vi "PopupViewLastErrorMessage.vi"() -> ()   [LabVIEW 2010]
uses:
  030 - EVENTS/03 - ToMessageHandlerProcess/enumMessageCriticity.ctl
  030 - EVENTS/EnumFgvEventCommand.ctl
  090 - ERRORS/Ctrls/enumLogAndView.ctl
  030 - EVENTS/03 - ToMessageHandlerProcess/ToMessageHandlerEvent.ctl
  030 - EVENTS/02 - ToScreens/ToScreensCommand.ctl
panel:
  out "Logo 600 X 200":picture
  out "Message":string
  out "Emitter":string caption="Emetteur"
  out "Date/Time":string caption="Date / Heure"
  out "Criticity":T1 caption="Criticité"
  in  "StringParam":string
  in  "bouton_quitter":bool
  # "Détail du message"
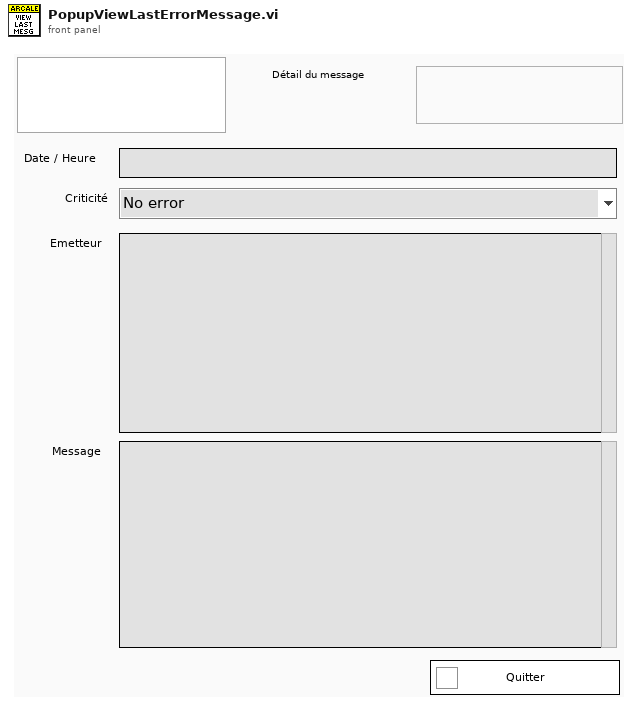
[diagram p1: front panel]
types:
  T1 = typedef "enumMessageCriticity.ctl" = enum16{"No error", "Info", "Warning", "Error", "Fatal error"}
  T2 = typedef "enumLogAndView.ctl" = enum16{"Log only", "Log and view"}
  T3 = typedef "EnumFgvEventCommand.ctl" = enum16{"Setup", "Cleanup", "Get"}
  T4 = typedef "ToMessageHandlerEvent.ctl" = cluster{"date / time":timestamp, "Criticity":T1, "Emitter":string, "Message":string}
  T5 = typedef "ApplicationInfos.ctl" = cluster{"ApplicationName":string, "ApplicationVersion":string, "Logo 600X200 path":path, "Logo 400X400 path":path, "Client":string}
  T6 = typedef "ToScreensCommand.ctl" = enum16{"Stop screen", "Stop all screens"}
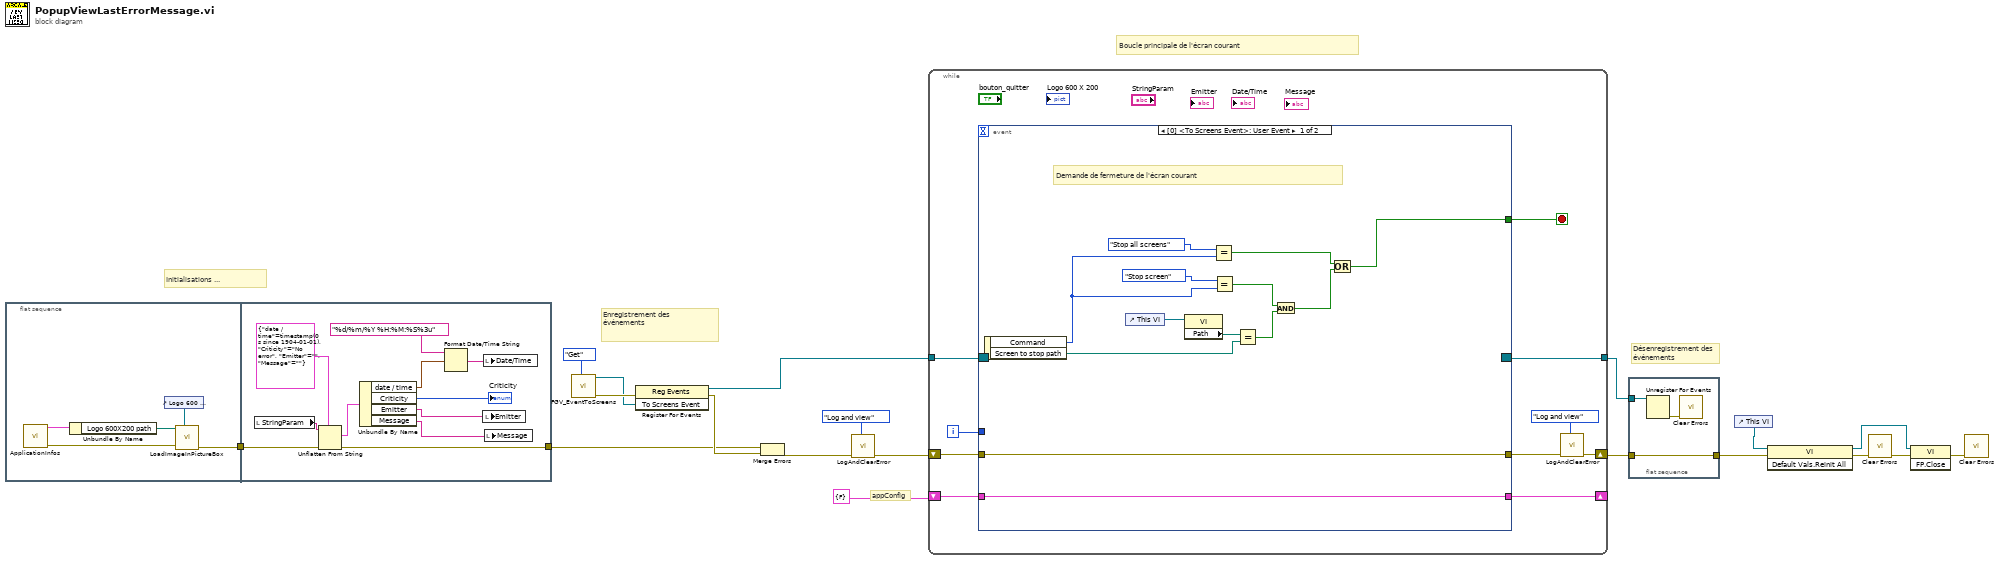
[diagram p0: block diagram]
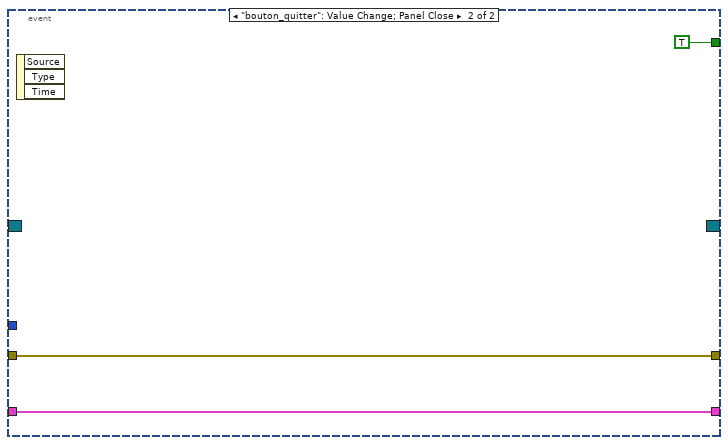
[diagram p2: hidden frame]
diagram:
  # "Initialisations ..."
  # "Boucle principale de l'écran courant"
  # "appConfig"
  # "Désenregistrement des \névénements"
  # "Enregistrement des \névénements"
  n1 = flat-sequence {
    tunnel: [w20] -> w8
    tunnel: w8 -> [w34]
    tunnel: [w33] -> w12
    frame #0 {
      n2 = call "ApplicationInfos.vi"() -> ("error out"=w24:errorcluster, "ApplicationInfo"=w22:T5)  [unwired: 10 in]
      n3 = Unbundle By Name(w22) -> ("Logo 600X200 path"=w21:path)
      n4 = control-ref of="Logo 600 X 200"() -> (w23:refnum<vi>)
      n5 = call "LoadImageInPictureBox.vi"("Pict Refnum In"=w23, "error in (no error)"=w24, "Image file path"=w21) -> ("error out"=w20:errorcluster)  [unwired: 8 in]
    }
    frame #1 {
      n6 = local read "StringParam"() -> (w35:string)
      n7 = Unflatten From String(type=T4 {"date / time"=timestamp(0 s since 1904-01-01), "Criticity"=enum."No error", "Emitter"="", "Message"=""} ("To message handler event"), binary string=w35, error in (no error)=w34) -> (value=w31:T4, error out=w33:errorcluster)  [unwired: 2 in, 1 out]
      n8 = Unbundle By Name(w31) -> ("date / time"=w27:timestamp, "Criticity"=→"Criticity":T1, "Emitter"=w28:string, "Message"=w29:string)
      n9 = Format Date/Time String(time format string (%c)="%d/%m/%Y %H:%M:%S%3u", seconds (now)=w27) -> (date/time string=w26:string)  [unwired: 1 in]
      n10 = local write "Emitter"(w28) -> ()
      n11 = local write "Date/Time"(w26) -> ()
      n12 = local write "Message"(w29) -> ()
    }
  }
  n13 = call "FGV_EventToScreens.vi"("Command"=EnumFgvEventCommand."Get") -> ("error out"=w16:errorcluster, "To Screens Event"=w14:refnum<user-event>)  [unwired: 9 in]
  n14 = register-events(error in=w16, w14) -> (reference out=w19:refnum<event-registration>, error out=w13:errorcluster)  [unwired: 1 in]
  n15 = Merge Errors(w12, w13) -> (w6:errorcluster)
  n16 = call "LogAndClearError.vi"("Log and view ?"=enumLogAndView."Log and view", "error in (no error)"=w6) -> ("error out"=w5:errorcluster)  [unwired: 9 in]
  n17 = while {
    tunnel: w19 -> [w45]
    shift-right: [w37] -> w11
    shift-left: w5 -> [w44]
    tunnel: [w43] -> w9
    shift-right: [w41] -> _
    shift-left: cluster{"Boolean":bool} {"Boolean"=FALSE} ("appConfig") -> [w42]
    i -> [w39]
    stop <- w40 stop-if-true
    n18 = event shown="[0] <To Screens Event>: User Event" {
      selector: w45 -> [_ _]
      dyn-events: [_ _] -> w43
      timeout: _ -> [_ _]
      tunnel: [w47 TRUE ("stopCurrentScreen")] -> w40
      tunnel: w44 -> [w46 w59]
      tunnel: [w46 w59] -> w38
      tunnel: w42 -> [w58 w60]
      tunnel: [w58 w60] -> w41
      tunnel: w39 -> [_ _]
      event User Event {
        # "Demande de fermeture de l'écran courant"
        n19 = event-data() -> ("Command"=w55:T6, "Screen to stop path"=w52:path)  [unwired: 1 out]
        n20 = control-ref of="This VI"() -> (w54:refnum<vi>)
        n21 = property class="VI"(reference=w54) -> ("Path"=w53:path)  [unwired: 1 in, 2 out]
        n22 = Equal?(x=ToScreensCommand."Stop all screens", y=w55) -> (x = y?=w49:bool)
        n23 = Equal?(x=ToScreensCommand."Stop screen", y=w55) -> (x = y?=w51:bool)
        n24 = Equal?(x=w53, y=w52) -> (x = y?=w50:bool)
        n25 = And(x=w51, y=w50) -> (x .and. y?=w48:bool)
        n26 = Or(x=w49, y=w48) -> (x .or. y?=w47:bool)
      }
      event "bouton_quitter": Value Change; Panel Close {
        n27 = event-data() -> ()  [unwired: 4 out]
      }
    }
    n28 = call "LogAndClearError.vi"("Log and view ?"=enumLogAndView."Log and view", "error in (no error)"=w38) -> ("error out"=w37:errorcluster)  [unwired: 9 in]
  }
  n29 = flat-sequence {
    tunnel: w9 -> [w64]
    tunnel: w11 -> [w62]
    tunnel: [w62] -> w10
    frame #0 {
      n30 = Unregister For Events(event registration refnum=w64) -> (error out=w63:errorcluster)  [unwired: 1 in]
      n31 = call <vilib>:"Clear Errors.vi"("error in (no error)"=w63) -> ()  [unwired: 7 out]
    }
  }
  n32 = control-ref of="This VI"() -> (w1:refnum<vi>)
  n33 = invoke class="VI" method="Default Vals.Reinit All"(reference=w1, error in=w10) -> (reference out=w2:refnum<vi>, error out=w17:errorcluster)  [unwired: 1 in, 1 out]
  n34 = call <vilib>:"Clear Errors.vi"("error in (no error)"=w17) -> ("error out"=w3:errorcluster)  [unwired: 6 out]
  n35 = invoke class="VI" method="FP.Close"(reference=w2, error in=w3) -> (error out=w4:errorcluster)  [unwired: 1 in, 2 out]
  n36 = call <vilib>:"Clear Errors.vi"("error in (no error)"=w4) -> ()  [unwired: 7 out]
